vi "check network path availability.vi"(8 "error in":errorcluster, 11 "Network Path":path) -> (0 "error out":errorcluster, 3 "base path":path)   [LabVIEW 2018]
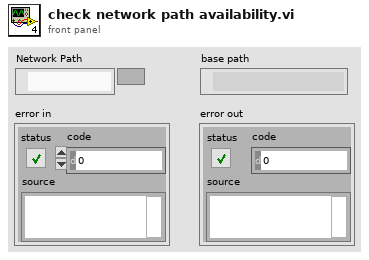
[diagram p1: front panel]
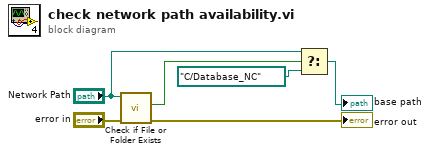
[diagram p0: block diagram]
diagram:
  n1 = call <vilib>:"Check if File or Folder Exists.vi"("error in (no error)"="error in", "path"="Network Path") -> ("error out"=→"error out":errorcluster, "file or folder exists?"=w2:bool)  [unwired: 7 in, 1 out]
  n2 = Select(t="Network Path", s=w2, f=path "C:/Database_NC") -> (s? t:f=→"base path":path)
